vi "sub-Language load.vi"(8 "error in (no error)":errorcluster caption="错误输入（无错误）", 10 "selected":i32, 11 "languages":cluster{string, "appended path":path, string}[](array[cluster])) -> (0 "error out":errorcluster caption="错误输出")   [LabVIEW 2011]
uses:
  <vilib>/Utility/config.llb/Read Key (String).vi
  <vilib>/Utility/config.llb/NI_LVConfig.lvlib
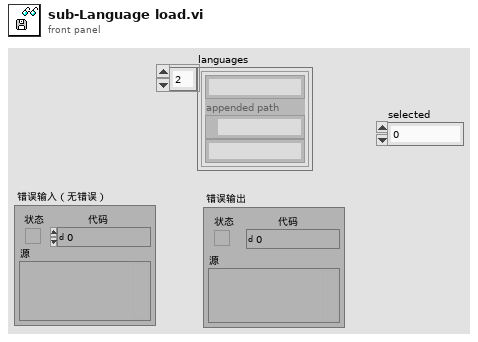
[diagram p1: front panel]
types:
  T1 = typedef "NI_LVConfig.lvlib/Config Data RefNum.ctl" = refnum<k1>
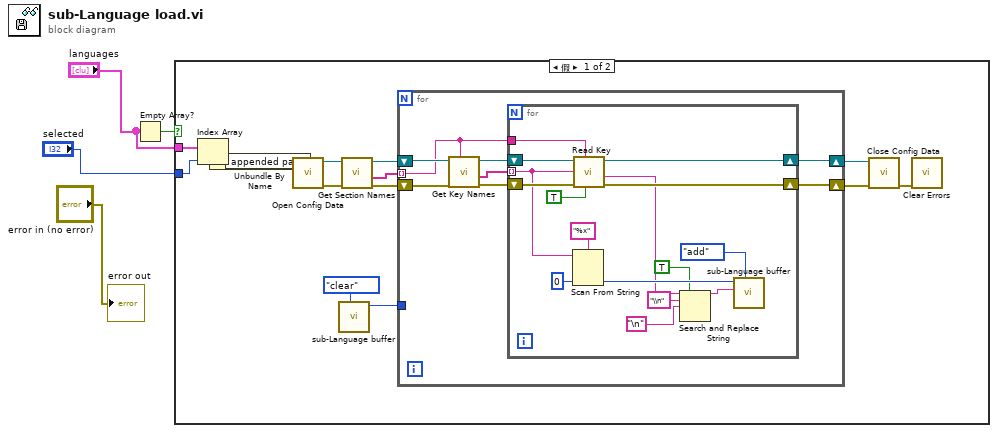
[diagram p0: block diagram]
diagram:
  n1 = Empty Array?(array="languages") -> (empty?=w4:bool)
  n2 = case shown="假" w4 {
    tunnel: "selected" -> [w5 _]
    tunnel: "languages" -> [w6 _]
    frame False {
      n3 = Index Array(array=w6, index=w5) -> (element=w18:cluster{string, "appended path":path, string})
      n4 = Unbundle By Name(w18) -> ("appended path"=w17:path)
      n5 = call <vilib>:"Open Config Data.vi"("configuration file path"=w17) -> ("error out"=w16:errorcluster, "refnum"=w15:T1)  [unwired: 8 in, 1 out]
      n6 = call "sub-Language buffer.vi"("operation"=enum16{"clear", "add", "get"}."clear") -> ("ID out"=w10:u32)  [unwired: 9 in, 1 out]
      n7 = call <vilib>:"Get Section Names.vi"("error in (no error)"=w16, "refnum"=w15) -> ("error out"=w12:errorcluster, "section names"=w13:string[], "refnum out"=w14:T1)  [unwired: 7 in]
      n8 = for {
        tunnel: w13 -> [w21] mode=indexing
        shift-right: [w19] -> w9
        shift-left: w12 -> [w25]
        shift-right: [w20] -> w8
        shift-left: w14 -> [w26]
        tunnel: w10 -> [_]
        n9 = call <vilib>:"Get Key Names.vi"("section"=w21, "error in (no error)"=w25, "refnum"=w26) -> ("error out"=w23:errorcluster, "key names"=w22:string[], "refnum out"=w24:T1)  [unwired: 5 in, 1 out]
        n10 = for {
          shift-right: [w36] -> w20
          shift-left: w24 -> [w42]
          shift-right: [w35] -> w19
          shift-left: w23 -> [w41]
          tunnel: w22 -> [w39] mode=indexing
          tunnel: w21 -> [w40]
          n11 = Scan From String(format string="%x" ("格式字符串"), input string=w39, default 1=u32 0 ("默认值 1")) -> (output 1=w34:u32)  [unwired: 2 in, 3 out]
          n12 = call-poly <vilib>:"Read Key.vi"("read raw string? (F)"=TRUE, "section"=w40, "error in (no error)"=w41, "key"=w39, "refnum"=w42) -> ("error out"=w35:errorcluster, "value"=w31:string, "refnum out"=w36:T1)  [unwired: 3 in, 1 out]
          n13 = Search and Replace String(replace all?=TRUE ("替换全部？(F)"), input string=w31, search string="\\n" ("搜索字符串"), replace string="\n") -> (result string=w27:string)  [unwired: 4 in, 3 out]
          n14 = call "sub-Language buffer.vi"("operation"=enum16{"clear", "add", "get"}."add", "str"=w27, "ID"=w34) -> ()  [unwired: 7 in, 2 out]
        }
      }
      n15 = call <vilib>:"Close Config Data.vi"("error in (no error)"=w9, "refnum"=w8) -> ("error out"=w7:errorcluster)  [unwired: 8 in, 1 out]
      n16 = call <vilib>:"Clear Errors.vi"("error in (no error)"=w7) -> ()  [unwired: 6 in, 1 out]
    }
    frame True {
    }
  }
  "error out" <- "error in (no error)"
